vi "GetTerminals.vi"(8 "error in":errorcluster, 11 "Node in":refnum<class "Node.lvclass">) -> (0 "error out":errorcluster, 3 "Node out":refnum<class "Node.lvclass">)   [LabVIEW 2014, in "Raspberry Pi Compatible Compiler for LabVIEW.lvlib" / "Node.lvclass"]
uses:
  Node.lvclass
  <vilib>/Utility/VariantDataType/Type.ctl
  Terminal/Terminal.lvclass
  <vilib>/Utility/VariantDataType/VariantType.lvlib
panel:
  out "Array":T1[](array[typedef])
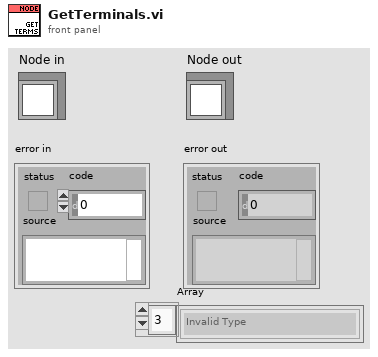
[diagram p1: front panel]
types:
  T1 = typedef "VariantType.lvlib/Type.ctl" = enum8{"Invalid Type", "Void", "I8", "I16", "I32", "I64", "U8", "U16", "U32", "U64", "Single Float", "Double Float", "Extended Float", "Single Complex", "Double Complex", "Extended Complex", "Enum U8", "Enum U16", "Enum U32", "Enum U64", "Single Float With Unit", "Double Float With Unit", "Extended Float With Unit", "Single Complex with Unit", "Double Complex with Unit", "Extended Complex with Unit", "Boolean", "String", "Path", "Picture", "Tag", "Array", "Cluster", "Variant", "LV Variant", "Waveform", "Timestamp", "Digital Waveform", "Digital Data", "ExpressData", "Refnum", "External Data", "VI", "Poly VI", "LabVIEW Class Instance", "Fixed Point"}
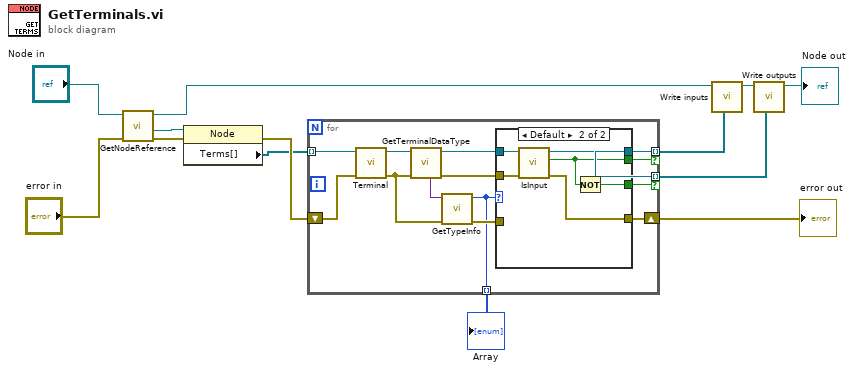
[diagram p0: block diagram]
diagram:
  n1 = call "GetNodeReference.vi"("error in"="error in", "Node in"="Node in") -> ("error out"=w8:errorcluster, "reference out"=w9:refnum<vi>, "Node out"=w5:refnum<class "Node.lvclass">)  [unwired: 7 in]
  n2 = property class="Node"(reference=w9, error in=w8) -> (error out=w12:errorcluster, "Terms[]"=w11:refnum<vi>[])  [unwired: 1 out]
  n3 = for {
    tunnel: w11 -> [w25] mode=indexing
    shift-right: [w24] -> w13
    shift-left: w12 -> [w26]
    tunnel: [w23] -> w6 mode=indexing if=w21
    tunnel: [w23] -> w2 mode=indexing if=w22
    tunnel: [w14] -> w1 mode=indexing
    n4 = call "Terminal.vi"("error in"=w26, "refnum"=w25) -> ("error out"=w16:errorcluster, "terminal"=w20:refnum<class "Terminal.lvclass">)  [unwired: 8 in]
    n5 = call "GetTerminalDataType.vi"("error in"=w16, "Terminal in"=w20) -> ("error out"=w18:errorcluster, "Terminal out"=w19:refnum<class "Terminal.lvclass">, "Data Type"=w17:variant)  [unwired: 5 in]
    n6 = call <vilib>:"GetTypeInfo.vi"("error in (no error)"=w16, "Variant"=w17) -> ("error out"=w15:errorcluster, "Type Enum"=w14:T1)  [unwired: 5 in, 3 out]
    n7 = case shown="Default" w14 {
      tunnel: [w27 w34] -> w24
      tunnel: [w28 w33] -> w23
      tunnel: [_ w32] -> w22
      tunnel: [_ w31] -> w21
      tunnel: w19 -> [w28 w30]
      tunnel: w18 -> [w27 w29]
      tunnel: w15 -> [_ _]
      frame "Void" {
      }
      frame Default {
        n8 = call-dynamic "IsInput.vi"("error in"=w29, "Terminal in"=w30) -> ("error out"=w34:errorcluster, "input"=w31:bool, "Terminal out"=w33:refnum<class "Terminal.lvclass">)  [unwired: 5 in]
        n9 = Not(x=w31) -> (.not. x?=w32:bool)
      }
    }
  }
  "error out" <- w13
  "Array" <- w1
  n10 = call-dynamic "Write inputs.vi"("inputs"=w6, "Node in"=w5) -> ("Node out"=w4:refnum<class "Node.lvclass">)  [unwired: 7 in]
  n11 = call-dynamic "Write outputs.vi"("outputs"=w2, "Node in"=w4) -> ("Node out"=→"Node out":refnum<class "Node.lvclass">)  [unwired: 7 in]
